vi "subsystem_checkCallbacks.vi"(8 "error in (no error)":errorcluster, 11 "ProgrammaticInitialization in":refnum<class "ProgrammaticInitialization.lvclass">) -> (0 "error out":errorcluster, 3 "ProgrammaticInitialization out":refnum<class "ProgrammaticInitialization.lvclass">)   [LabVIEW 2016, in "ProgrammaticInitialization.lvclass"]
uses:
  ProgrammaticInitialization.lvclass
  ProgrammaticInitialization.lvclass/ProgrammaticInitialization.ctl
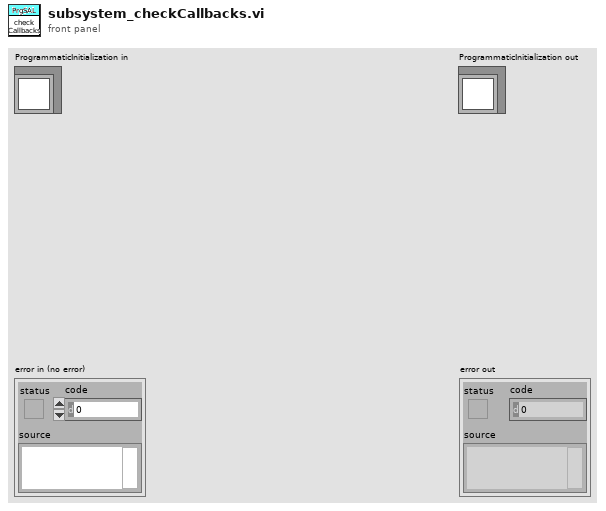
[diagram p1: front panel]
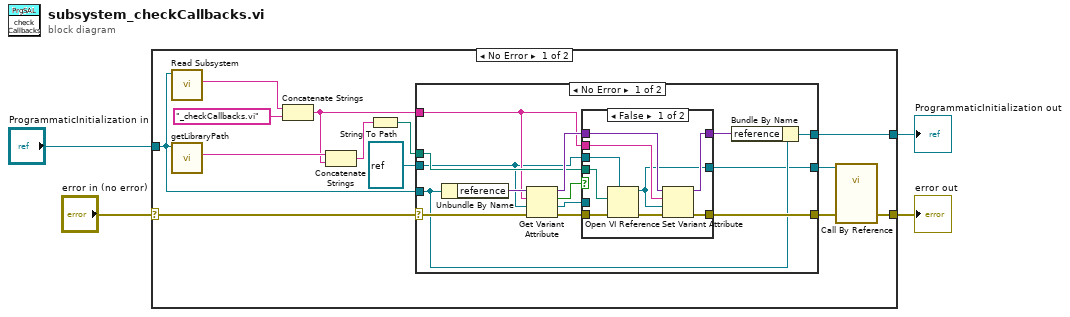
[diagram p0: block diagram]
diagram:
  n1 = case shown="No Error" "error in (no error)" {
    selector: "error in (no error)" -> [w11 w48]
    tunnel: [w15 w48] -> w3
    tunnel: [w13 w47] -> w1
    tunnel: "ProgrammaticInitialization in" -> [w14 w47]
    frame No Error {
      n2 = call-dynamic "Read Subsystem.vi"("ProgrammaticInitialization in"=w14) -> ("Subsystem"=w17:string)  [unwired: 8 in, 2 out]
      n3 = call "getLibraryPath.vi"("ProgrammaticInitialization in"=w14) -> ("SAL_Library"=w10:string)  [unwired: 8 in, 2 out]
      n4 = Concatenate Strings(w17, "_checkCallbacks.vi" ("string")) -> (w7:string)
      n5 = Concatenate Strings(w10, w7) -> (w8:string)
      n6 = String To Path(string=w8) -> (path=w9:path)
      n7 = case shown="No Error" w11 {
        selector: w11 -> [w28 w46]
        tunnel: [w27 w46] -> w6
        tunnel: [w23 w45] -> w13
        tunnel: w14 -> [w22 w45]
        tunnel: w7 -> [w20 _]
        tunnel: refnum<vi> refnum ("type specifier VI Refnum (for type only)") -> [w18 w44]
        tunnel: w9 -> [w21 _]
        tunnel: [w19 w44] -> w5
        frame No Error {
          n8 = Unbundle By Name(w22) -> ("reference"=w26:variant)
          n9 = Get Variant Attribute(Variant=w26, name=w20, default value (empty Variant)=w18, error in=w28) -> (duplicate Variant=w25:variant, found=w31:bool, value=w29:refnum<vi>, error out=w30:errorcluster)
          n10 = case shown="False" w31 {
            tunnel: w30 -> [w38 w43]
            tunnel: w29 -> [_ w41]
            tunnel: [w40 w43] -> w27
            tunnel: w25 -> [w33 w42]
            tunnel: [w39 w42] -> w24
            tunnel: w18 -> [w36 _]
            tunnel: w21 -> [w35 _]
            tunnel: w20 -> [w34 _]
            tunnel: [w32 w41] -> w19
            frame False {
              n11 = Open VI Reference(type specifier VI Refnum (for type only)=w36, vi path=w35, error in (no error)=w38) -> (vi reference=w32:refnum<vi>, error out=w37:errorcluster)  [unwired: 3 in]
              n12 = Set Variant Attribute(Variant=w33, name=w34, value=w32, error in=w37) -> (Variant out=w39:variant, error out=w40:errorcluster)  [unwired: 1 out]
            }
            frame True {
            }
          }
          n13 = Bundle By Name(cluster=w22, "reference"=w24) -> (w23:refnum<class "ProgrammaticInitialization.lvclass">)
        }
        frame Error {
        }
      }
      n14 = call-by-ref "?"(reference=w5, "error in (no error)"=w6) -> ("error out"=w15:errorcluster)  [unwired: 11 in, 2 out]
    }
    frame Error {
    }
  }
  "error out" <- w3
  "ProgrammaticInitialization out" <- w1
